vi "JSON_extract_Data_1 (SubVI).vi"(8 "data type":string[](array[string]), 11 "Response in":string) -> (2 "id":u8, 3 "Response out":string[](array[string]))   [LabVIEW 2015]
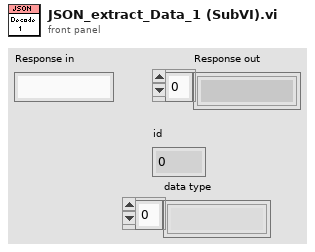
[diagram p1: front panel]
types:
  T1 = cluster{"type":string, "phase":string, "id":u8, "status":i32, "status_msg":string, "device":string, "data":string[]}
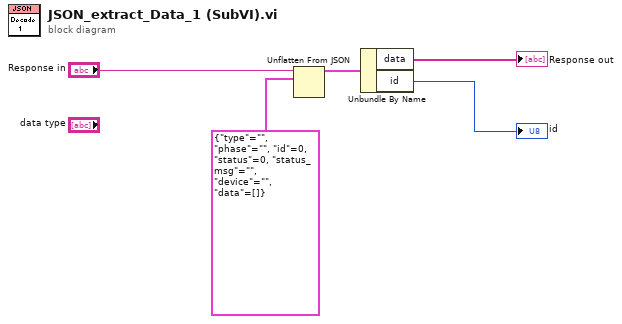
[diagram p0: block diagram]
diagram:
  n1 = Unflatten From JSON(JSON string="Response in", type and defaults=T1 {"type"="", "phase"="", "id"=0, "status"=0, "status_msg"="", "device"="", "data"=[]}) -> (value=w3:T1)  [unwired: 5 in, 1 out]
  n2 = Unbundle By Name(w3) -> ("data"=→"Response out":string[], "id"=→"id":u8)
